vi "Read Trigger Mode Attr.vi"(8 "error in (no error)":errorcluster, 11 "Camera Quick Settings Panel in":refnum<class "Camera Quick Settings Panel.lvclass">) -> (0 "error out":errorcluster, 2 "Trigger Mode Attr":string="CameraAttributes::AcquisitionTrigger::TriggerMode", 3 "Camera Quick Settings Panel out":refnum<class "Camera Quick Settings Panel.lvclass">)   [LabVIEW 2014, in "Camera Quick Settings Panel.lvlib" / "Camera Quick Settings Panel.lvclass"]
uses:
  Camera Quick Settings Panel.lvclass
  Camera Quick Settings Panel.lvclass/Camera Quick Settings Panel.ctl
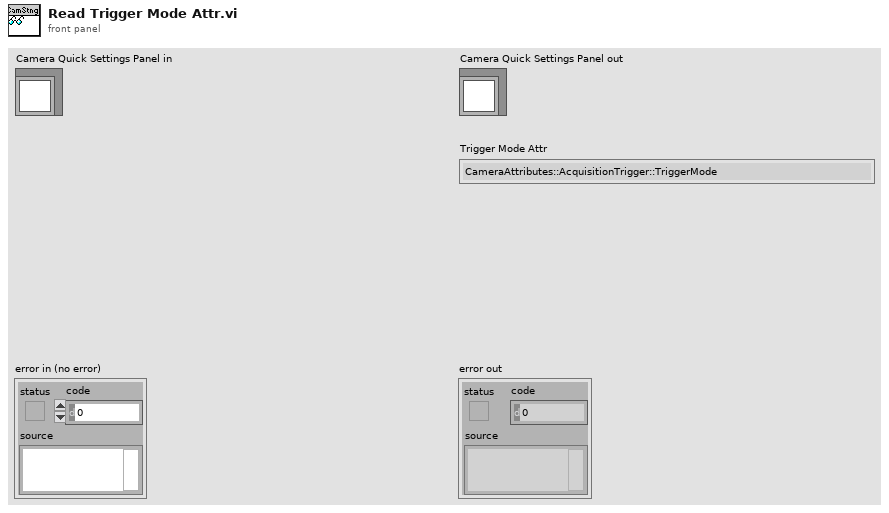
[diagram p1: front panel]
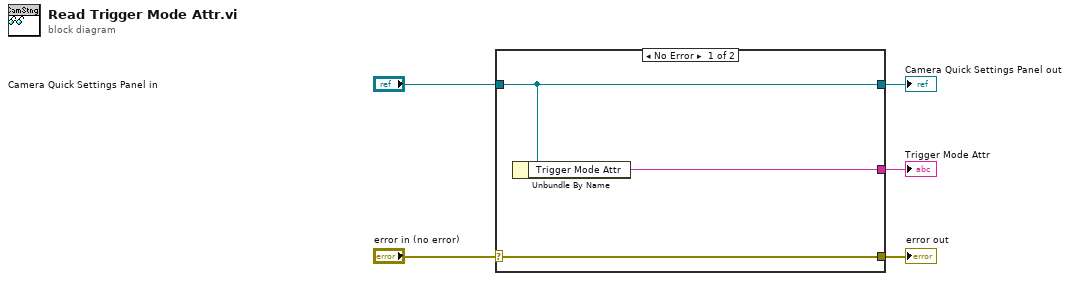
[diagram p0: block diagram]
diagram:
  n1 = case shown="No Error" "error in (no error)" {
    selector: "error in (no error)" -> [w8 w9]
    tunnel: [w8 w9] -> w4
    tunnel: [w7 w10] -> w2
    tunnel: "Camera Quick Settings Panel in" -> [w7 w10]
    tunnel: [w6 _] -> w1
    frame No Error {
      n2 = Unbundle By Name(w7) -> ("Trigger Mode Attr"=w6:string)
    }
    frame Error {
    }
  }
  "error out" <- w4
  "Camera Quick Settings Panel out" <- w2
  "Trigger Mode Attr" <- w1
